vi "LimitHeightWidthByMinimum.vi"(10 "Minimal":cluster{"Width":i32, "Height":i32}, 11 "Height Width in":cluster{"Width":i32, "Height":i32}) -> (3 "Limited Height Width out":T1)   [LabVIEW 2022 SP3, in "PentaPanesLibrary.lvlib" / "PentaPanes.lvclass"]
uses:
  PentaPanes.lvclass
  <vilib>/Utility/miscctls.llb/LVBoundsTypeDef.ctl
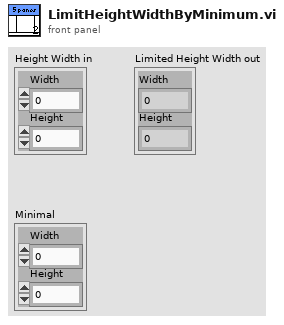
[diagram p1: front panel]
types:
  T1 = typedef "LVBoundsTypeDef.ctl" = cluster{"Width":i32, "Height":i32}
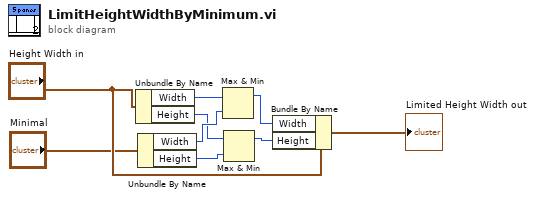
[diagram p0: block diagram]
diagram:
  n1 = Unbundle By Name("Height Width in") -> ("Width"=w5:i32, "Height"=w1:i32)
  n2 = Unbundle By Name("Minimal") -> ("Width"=w6:i32, "Height"=w2:i32)
  n3 = Max & Min(x=w5, y=w6) -> (max(x,y)=w7:i32)  [unwired: 1 out]
  n4 = Max & Min(x=w1, y=w2) -> (max(x,y)=w8:i32)  [unwired: 1 out]
  n5 = Bundle By Name(cluster="Height Width in", "Width"=w7, "Height"=w8) -> (→"Limited Height Width out":cluster{"Width":i32, "Height":i32})
